vi "fibonacci.vi"() -> ()   [LabVIEW 2019]
panel:
  out "Array 2":string[][](array[string])
  out "Array":string[][](array[string])
  in  "Numeric":i32
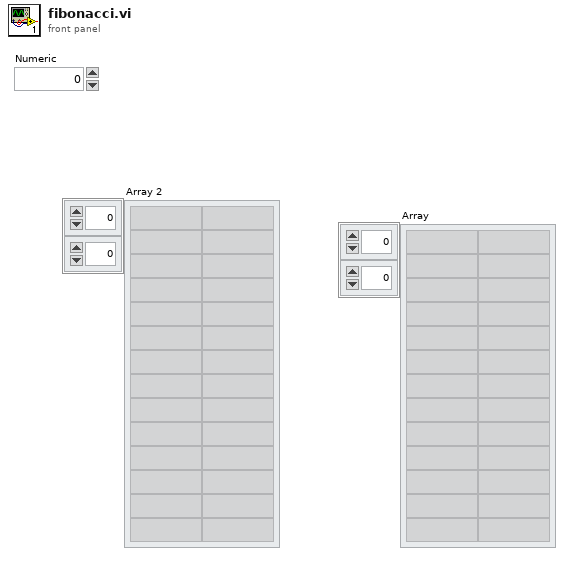
[diagram p1: front panel]
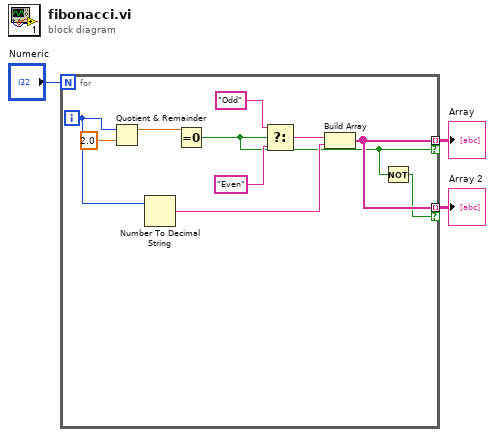
[diagram p0: block diagram]
diagram:
  n1 = for {
    N: "Numeric" -> [_]
    tunnel: [w6] -> w2 mode=indexing if=w5
    tunnel: [w6] -> w1 mode=indexing if=w4
    i -> [w8]
    n2 = Quotient & Remainder(x=w8, y=2.0) -> (x-y*floor(x/y)=w12:dbl)  [unwired: 1 out]
    n3 = Number To Decimal String(number=w8) -> (decimal integer string=w7:string)  [unwired: 1 in]
    n4 = Equal To 0?(x=w12) -> (x = 0?=w5:bool)
    n5 = Select(t="Odd", s=w5, f="Even") -> (s? t:f=w9:string)
    n6 = Build Array(w9, w7) -> (w6:string[])
    n7 = Not(x=w5) -> (.not. x?=w4:bool)
  }
  "Array" <- w2
  "Array 2" <- w1
